vi "Overlay X.vi"(11 "Refnum in":T1) -> (3 "Refnum out":T1)   [LabVIEW 2015]
uses:
  <vilib>/vision/Image Controls.llb/IMAQ Image.ctl
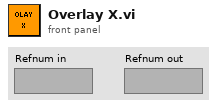
[diagram p1: front panel]
types:
  T1 = typedef "IMAQ Image.ctl" = refnum<image>
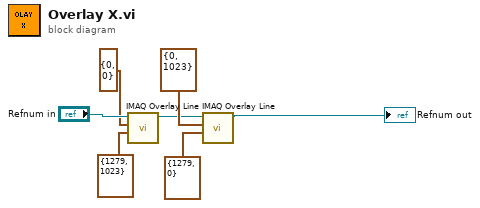
[diagram p0: block diagram]
diagram:
  n1 = call "IMAQ Overlay Line"("End Point"=cluster{"X":i32, "Y":i32} {"X"=1279, "Y"=1023}, "Start Point"=cluster{"X":i32, "Y":i32} {"X"=0, "Y"=0}, "Image"="Refnum in") -> ("Image Out"=w1:T1)  [unwired: 7 in, 1 out]
  n2 = call "IMAQ Overlay Line"("End Point"=cluster{"X":i32, "Y":i32} {"X"=1279, "Y"=0}, "Start Point"=cluster{"X":i32, "Y":i32} {"X"=0, "Y"=1023} ("End Point"), "Image"=w1) -> ("Image Out"=→"Refnum out":T1)  [unwired: 7 in, 1 out]
